vi "SmallestAngle.vi"(10 "Angle B":dbl, 11 "Angle A":dbl) -> (3 "Smallest B to A":dbl)   [LabVIEW 2016]
doc: "Returns the smallest angle from B to A"
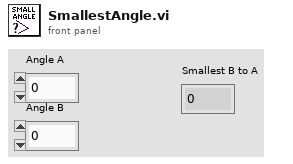
[diagram p1: front panel]
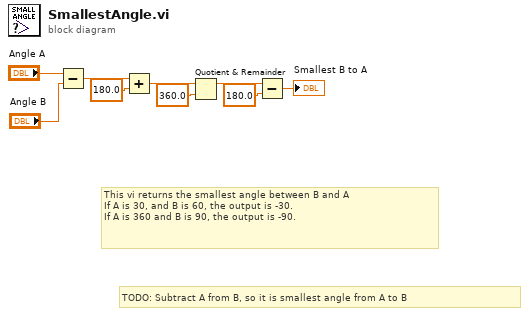
[diagram p0: block diagram]
diagram:
  # "TODO: Subtract A from B, so it is smallest angle from A to B"
  # "This vi returns the smallest angle between B and A\nIf A is 30, and B is 60, the output is -30.\nIf A is 360 and B is 90, the output is -90."
  n1 = Subtract(x="Angle A", y="Angle B") -> (x-y=w7:dbl)
  n2 = Add(x=w7, y=180.0) -> (x+y=w5:dbl)
  n3 = Quotient & Remainder(x=w5, y=360.0) -> (x-y*floor(x/y)=w3:dbl)  [unwired: 1 out]
  n4 = Subtract(x=w3, y=180.0) -> (x-y=→"Smallest B to A":dbl)
